vi "Get_devices_information.vi"(8 "error in (no error)":errorcluster, 11 "Dali_usb_tridonics in":refnum<class "Dali_usb_tridonics.lvclass">) -> (0 "error out":errorcluster, 2 "devices_found":i32, 3 "Dali_usb_tridonics out":refnum<class "Dali_usb_tridonics.lvclass">)   [LabVIEW 2014, in "Driver_interaction.lvlib" / "Dali_usb_tridonics.lvclass"]
uses:
  Dali_usb_tridonics.lvclass
  Dali_usb_tridonics.lvclass/Dali_usb_tridonics.ctl
  _Driver_interaction/_Driver_interaction.lvclass
  Vendor/Dali_usb.lvlib
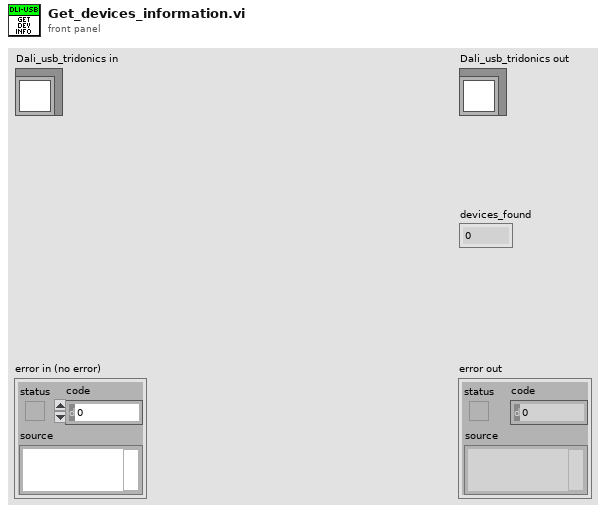
[diagram p1: front panel]
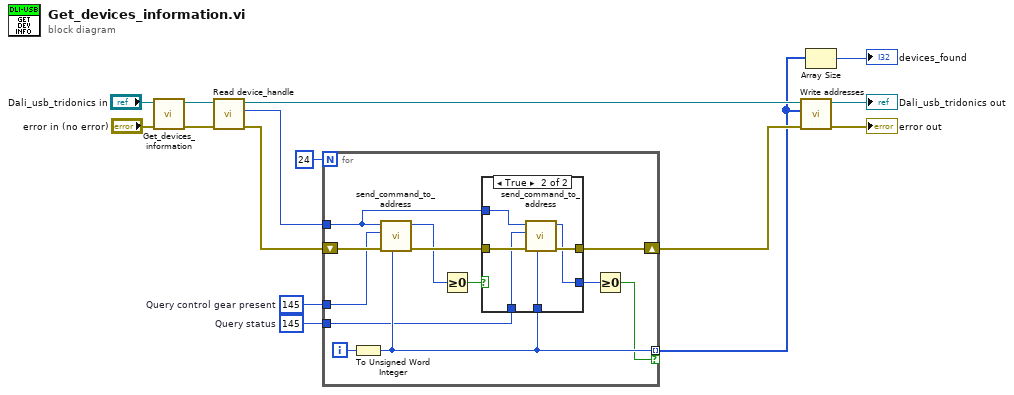
[diagram p0: block diagram]
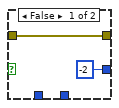
[diagram p2: hidden frame]
diagram:
  w8 = u32 145  # Query status
  w9 = u32 145  # Query control gear present
  n1 = call-parent "Get_devices_information.vi"("error in (no error)"="error in (no error)", "_Driver_interaction in"="Dali_usb_tridonics in") -> ("error out"=w13:errorcluster, "_Driver_interaction out"=w12:refnum<class "Dali_usb_tridonics.lvclass">)  [unwired: 7 in, 1 out]
  n2 = call "Read device_handle.vi"("error in (no error)"=w13, "Dali_usb_tridonics in"=w12) -> ("error out"=w4:errorcluster, "device_handle"=w11:i32, "Dali_usb_tridonics out"=w7:refnum<class "Dali_usb_tridonics.lvclass">)  [unwired: 7 in]
  n3 = for {
    N: 24 -> [_]
    shift-right: [w22] -> w3
    shift-left: w4 -> [w27]
    tunnel: w11 -> [w25]
    tunnel: [w23] -> w2 mode=indexing if=w16
    tunnel: w9 -> [w21]
    tunnel: w8 -> [w20]
    i -> [w24]
    n4 = To Unsigned Word Integer(number=w24) -> (unsigned 16bit integer=w23:u16)
    n5 = call "send_command_to_address.vi"("Address"=w23, "error in (no error)"=w27, "command"=w21, "device_handle"=w25) -> ("error out"=w26:errorcluster, "response_command"=w19:i32)  [unwired: 4 in, 2 out]
    n6 = Greater Or Equal To 0?(x=w19) -> (x >= 0?=w18:bool)
    n7 = case shown="True" w18 {
      tunnel: w26 -> [w29 w35]
      tunnel: w25 -> [_ w34]
      tunnel: w23 -> [_ w33]
      tunnel: [w29 w32] -> w22
      tunnel: w20 -> [_ w31]
      tunnel: [-2 ("response_command") w30] -> w17
      frame False {
      }
      frame True {
        n8 = call "send_command_to_address.vi"("Address"=w33, "error in (no error)"=w35, "command"=w31, "device_handle"=w34) -> ("error out"=w32:errorcluster, "response_command"=w30:i32)  [unwired: 4 in, 2 out]
      }
    }
    n9 = Greater Or Equal To 0?(x=w17) -> (x >= 0?=w16:bool)
  }
  n10 = call "Write addresses.vi"("error in (no error)"=w3, "addresses"=w2, "Dali_usb_tridonics in"=w7) -> ("error out"=→"error out":errorcluster, "Dali_usb_tridonics out"=→"Dali_usb_tridonics out":refnum<class "Dali_usb_tridonics.lvclass">)  [unwired: 7 in]
  n11 = Array Size(array=w2) -> (size(s)=→"devices_found":i32)
